vi "setSweepConfiguration.vi"(8 "error in (no error)":errorcluster, 10 "Configure Sweep":T1 {"Sweep IV Step (V)" format="%#_6p"; "Sweep End (V)" format="%#_6p"; "Sweep Start (V)" format="%#_6p"; "Sweep Lockin Time (s)" format="%#_6p"}, 11 "Instrument.Lockin in":refnum<class "Instrument.Lockin.lvclass">) -> (0 "error out":errorcluster, 3 "Instrument.Lockin out":refnum<class "Instrument.Lockin.lvclass">)   [LabVIEW 2016, in "Instrument.Lockin.lvclass"]
doc: "API to put lockin into remote mode.\n\nIf address=\"\", this API reads from localhost\nIf address is remote lockin, you need to add this computer to allowed whitelist on the lockin computer you are trying to access."
uses:
  Instrument.Lockin.lvclass
  LockinDAQ/Typedefs/Sweep Configuration--Cluster.ctl
  Typedefs/Instrument.Lockin.Commands--Enum.ctl
  LockinDAQ/LockinDAQ.lvclass
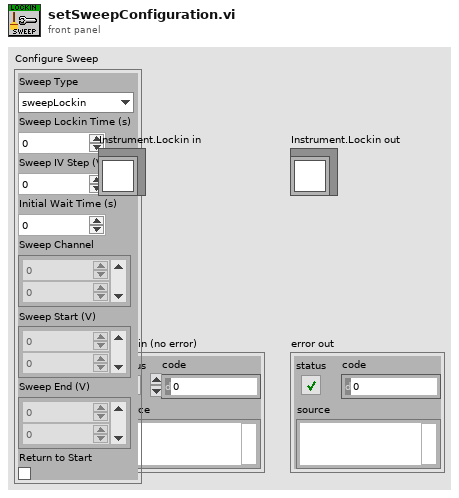
[diagram p1: front panel]
types:
  T1 = typedef "LockinDAQ.lvclass/Sweep Configuration--Cluster.ctl" = cluster{"Sweep Type":enum16{"sweepLockin", "sweepIV"}, "Sweep Lockin Time (s)":dbl, "Sweep IV Step (V)":dbl, "Initial Wait Time (s)":dbl, "Sweep Channel":i32[], "Sweep Start (V)":dbl[], "Sweep End (V)":dbl[], "Return to Start":bool}
  T2 = typedef "Instrument.Lockin.lvclass/Instrument.Lockin.Commands--Enum.ctl" = enum16{"setAO", "setAO_Amplitude", "setAO_DC", "setAO_Frequency", "setAO_Phase", "setAO_Function", "setAO_I+", "setREF", "setREF_Frequency", "setREF_Phase", "setIVmode", "Reset", "setSampling", "Trigger", "getAO", "getAI", "getResults", "getTrigger", "getIVmode", "getSampling", "getAOconfig", "getREFconfig", "setGain", "getGain", "setAutoSampling", "getAutoSampling", "setSweep", "getStatus", "getSweepResults", "getIVSweepResults", "startSweep", "stopSweep", "setAUX", "getAUX"}
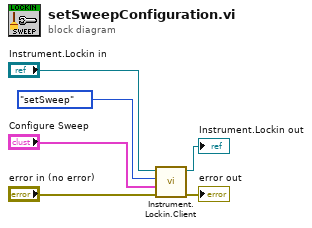
[diagram p0: block diagram]
diagram:
  n1 = call "Instrument.Lockin.Client.vi"("error in (no error)"="error in (no error)", "Data"="Configure Sweep", "Command"=Instrument.Lockin.Commands--Enum."setSweep", "Instrument.Lockin in"="Instrument.Lockin in") -> ("error out"=→"error out":errorcluster, "Instrument.Lockin out"=→"Instrument.Lockin out":refnum<class "Instrument.Lockin.lvclass">)  [unwired: 5 in, 1 out]
